vi "Position faisceau.vi"(0 "R1":dbl, 5 "R2":dbl, 7 "error in (no error)":T1 caption="entrée d'erreur (pas d'erreur)", 9 "Capteur 1":dbl[](array[numeric]), 11 "Capteur 2":dbl[](array[numeric])) -> (6 "Coord":dbl[](array[numeric]), 15 "error out":T1 caption="sortie d'erreur")   [LabVIEW 2018]
uses:
  <vilib>/imath/engines/lvmath2/RunTimeEngine/NodeEndStatement/NIMS_NodeEndStatement_Output.vi
  <instcachedir>/0/NIMS_NodeEndStatement_Output_53EC0D466D134D7ABD903AC30B43404B.lvgen/NIMS_NodeEndStatement_Output_53EC0D466D134D7ABD903AC30B43404B_001.vi
  <vilib>/imath/engines/lvmath2/RunTimeEngine/ErrorHandling/NIMS_Finalize Error.vi
  <instcachedir>/0/NIMS_NodeEndStatement_Output_53EC0D466D134D7ABD903AC30B43404B.lvgen/NIMS_NodeEndStatement_Output_53EC0D466D134D7ABD903AC30B43404B_009.vi
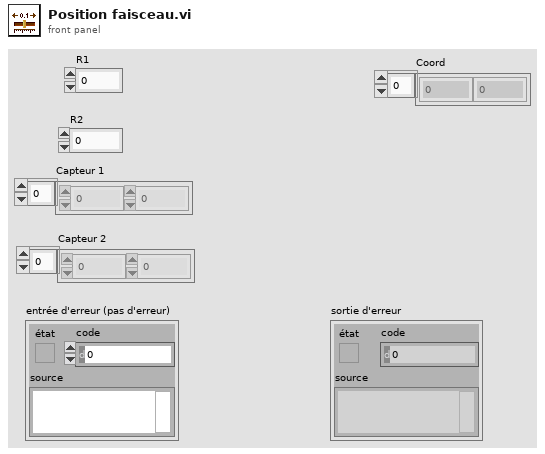
[diagram p1: front panel]
types:
  T1 = cluster{"état":bool, "code":i32, "source":string}
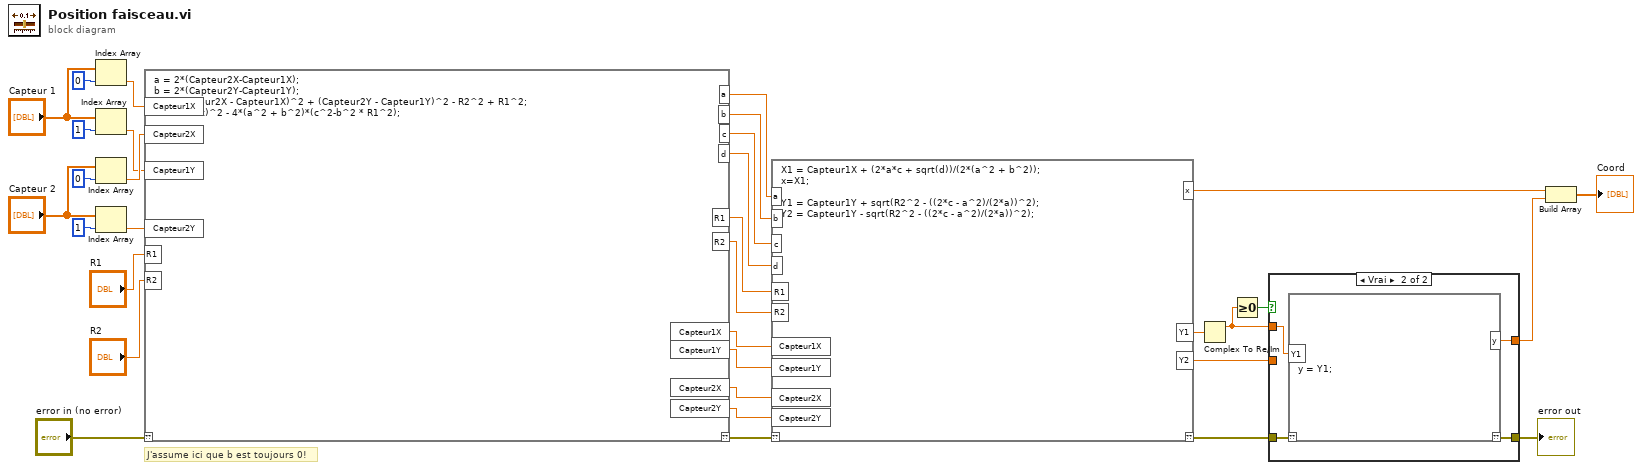
[diagram p0: block diagram]
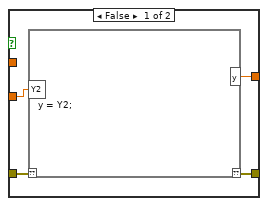
[diagram p2: hidden frame]
diagram:
  # "J'assume ici que b est toujours 0!"
  n1 = Index Array(array="Capteur 1", index=0) -> (element=w31:dbl)
  n2 = Index Array(array="Capteur 1", index=1) -> (element=w22:dbl)
  n3 = Index Array(array="Capteur 2", index=0) -> (element=w30:dbl)
  n4 = Index Array(array="Capteur 2", index=1) -> (element=w23:dbl)
  n5 = mathscript code="a = 2*(Capteur2X-Capteur1X);\nb = 2*(Capteur2Y-Capteur1Y);\nc = (Capteur2X - Capteur1X)^2 + (Capteur2Y - Capteur1Y)^2 - R2^2 + R1^2;\nd = (2*a*c)^2 - 4*(a^2 + b^2)*(c^2-b^2 * R1^2);"("??"="error in (no error)", "Capteur1X"=w31, "Capteur2X"=w30, "Capteur1Y"=w22, "Capteur2Y"=w23, "R1"="R1", "R2"="R2") -> ("??"=w10:errorcluster, "a"=w20:dbl, "b"=w19:dbl, "c"=w18:dbl, "d"=w17:dbl, "Capteur1X"=w14:dbl, "Capteur1Y"=w13:dbl, "Capteur2X"=w12:dbl, "Capteur2Y"=w11:dbl, "R1"=w16:dbl, "R2"=w15:dbl)
  n6 = mathscript code="X1 = Capteur1X + (2*a*c + sqrt(d))/(2*(a^2 + b^2));\nx=X1;\n\nY1 = Capteur1Y + sqrt(R2^2 - ((2*c - a^2)/(2*a))^2);\nY2 = Capteur1Y - sqrt(R2^2 - ((2*c - a^2)/(2*a))^2);"("??"=w10, "a"=w20, "b"=w19, "c"=w18, "d"=w17, "R1"=w16, "R2"=w15, "Capteur1X"=w14, "Capteur1Y"=w13, "Capteur2X"=w12, "Capteur2Y"=w11) -> ("??"=w5:errorcluster, "x"=w2:cdb, "Y1"=w9:cdb, "Y2"=w6:cdb)
  n7 = Complex To Re/Im(x + iy=w9) -> (x=w8:dbl)  [unwired: 1 out]
  n8 = Greater Or Equal To 0?(x=w8) -> (x >= 0?=w7:bool)
  n9 = case shown="Vrai" w7 {
    tunnel: w8 -> [_ w56]
    tunnel: w6 -> [w37 _]
    tunnel: w5 -> [w36 w55]
    tunnel: [w35 w54] -> w4
    tunnel: [w34 w53] -> w3
    frame False {
      n10 = mathscript code="y = Y2;"("??"=w36, "Y2"=w37) -> ("??"=w35:errorcluster, "y"=w34:cdb)
    }
    frame True {
      n11 = mathscript code="y = Y1;"("??"=w55, "Y1"=w56) -> ("??"=w54:errorcluster, "y"=w53:dbl)
    }
  }
  "error out" <- w4
  n12 = Build Array(w2, w3) -> (→"Coord":cdb[])
